vi "CSV_Setup_Data_Handler.vi"(0 "first iteration":bool, 1 "Timeout 1":bool, 7 "Sample Data":dbl[](array[numeric]), 9 "Sample Data 2":dbl[](array[numeric]), 11 "Data":T1={"Pinch-valve"="", "XLP 6000 Pump"="", "Camera1"="", "Camera2"="", "Img_Capt"=FALSE, "Actuator"=FALSE, "Pump"=FALSE, "Cam 1"=FALSE, "Cam 2"=FALSE, "Empty_Refill"=FALSE, "Crop"=FALSE, "Light intensity"=0, "Exposure Time"=0.0, "Sample Name"="", "Operator"="", "Calibration 1"=path "", "Calibration 2"=path "", "Framerate"=0, "Timeout Sample"=0, "Collection date"="", "Sample size threshold"=0, "Empty start"=0, "Command"="", "Station"="", "Species Name"="", "Other Notes"="", "Aperture"=enum."Item 0", "Image Process Queue Size"=0, "Image Save Queue Size"=0, "Overload threshold"=0, "Max Framerate"=0, "Rectangle 1"={"Left"=0, "Top"=0, "Right"=0, "Bottom"=0, "Rotation"=0.0}, "Rectangle 2"={"Left"=0, "Top"=100, "Right"=100, "Bottom"=0, "Rotation"=0.0}, "Detection Region %"=200.0, "Detect 1"=path "", "Detect 2"=path "", "Max large object threshold"=500, "Open(T)/Close(F)"=FALSE, "Img_Capt Begin"=FALSE, "Dispense Speed"=0, "Flush Size"=0, "Location"="", "Latitude"="", "Longitude"="", "Determiner"="", "Sex"="", "Camera1_Img"=refnum, "Camera2_Img"=refnum, "Img1_Orig_Disp"=refnum, "Img2_Orig_Disp"=refnum, "Img1_Orig_RGB"=refnum, "Img2_Orig_RGB"=refnum, "Blue_Plane_Extract"=refnum, "Subtracted_Plane"=refnum, "Img1_Binary"=refnum, "Img2_Binary"=refnum, "Crop_Mask"=refnum, "Img1_Save"=refnum, "Img2_Save"=refnum, "Img1_Cali_Full"=refnum, "Img2_Cali_Full"=refnum, "Img1_Cali_Detect"=refnum, "Img2_Cali_Detect"=refnum, "Cam 1 queue"=refnum, "Cam 2 queue"=refnum, "Cam 1 - save queue"=refnum, "Cam 2 - save queue"=refnum, "Overlay_Ring"=0, "SystemVersion"=0, "System Serial"="", "Legacy Cam Attributes"=FALSE, "Camera Orientation 1"="", "Camera Orientation 2"="", "Pixel to mm 1"=0.0, "Pixel to mm 2"=0.0, "CAM1 Model"=enum."a2A5328-15ucBAS", "CAM2 Model"=enum."a2A5328-15ucBAS", "Flush Insect"=FALSE, "Pump Size"=FALSE, "Barcode"="", "Phase3"=FALSE, "Mega F3"="", "Container nr."=0.0, "Flush Error"=TRUE, "Start System"=FALSE, "Size Interval"=0.0, "Mun. of containers"=0.0, "Sorting sys."=FALSE, "Initial size"=0.0} {"SystemVersion" items=["Standard", "XL"]; "Overlay_Ring" items=["Session Data", "Extended Setup", "Buffer", "Camera", "Dispenser", "Stats", "Connections"]; "Flush Size" min=1; "Dispense Speed" min=1; "Rectangle 2"."Rotation" format="%.2f"; "Rectangle 2"."Left" scale=0.0..1024.0; "Rectangle 2"."Right" scale=0.0..1024.0; "Rectangle 1"."Rotation" format="%.2f"; "Rectangle 1"."Left" scale=0.0..1024.0; "Rectangle 1"."Right" scale=0.0..1024.0; "Max Framerate" min=1; "Overload threshold" min=1; "Image Save Queue Size" min=1; "Image Process Queue Size" min=1; "Empty start" min=1; "Sample size threshold" min=1; "Framerate" min=1; "Light intensity" scale=0.0..100.0}, 12 "Timeout 2":bool) -> (4 "Sample Name":string, 6 "Ready file created":bool, 10 "Cam1_Stats":cluster{"Mean_Area":i32, "Img_Count":u32} caption="Camera 1", 14 "Container barcode":string, 15 "Cam2_Stats":cluster{"Mean_Area":i32, "Img_Count":u32} caption="Camera 2")   [LabVIEW 2024]
uses:
  controls/Data.ctl
  <vilib>/userDefined/High Color/IMAQdx.ctl
  <vilib>/vision/Image Controls.llb/IMAQ Image.ctl
panel:
  in  "Stop":bool
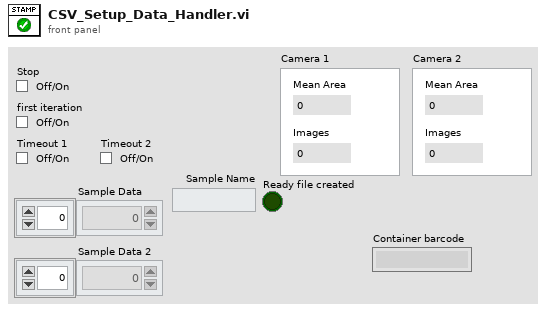
[diagram p1: front panel]
types:
  T1 = typedef "Data.ctl" = cluster{"Pinch-valve":refnum<visa-resource-name>, "XLP 6000 Pump":refnum<visa-resource-name>, "Camera1":T2, "Camera2":T2, "Img_Capt":bool, "Actuator":bool, "Pump":bool, "Cam 1":bool, "Cam 2":bool, "Empty_Refill":bool, "Crop":bool, "Light intensity":i32, "Exposure Time":dbl, "Sample Name":string, "Operator":string, "Calibration 1":path, "Calibration 2":path, "Framerate":i32, "Timeout Sample":i32, "Collection date":string, "Sample size threshold":i32, "Empty start":u32, "Command":string, "Station":string, "Species Name":string, "Other Notes":string, "Aperture":enum32{"Item 0", "Item 1", "Item 2", "Item 3"}, "Image Process Queue Size":i32, "Image Save Queue Size":i32, "Overload threshold":i32, "Max Framerate":i32, "Rectangle 1":T3, "Rectangle 2":T3, "Detection Region %":dbl, "Detect 1":path, "Detect 2":path, "Max large object threshold":i32, "Open(T)/Close(F)":bool, "Img_Capt Begin":bool, "Dispense Speed":i32, "Flush Size":i32, "Location":string, "Latitude":string, "Longitude":string, "Determiner":string, "Sex":string, "Camera1_Img":T4, "Camera2_Img":T4, "Img1_Orig_Disp":T4, "Img2_Orig_Disp":T4, "Img1_Orig_RGB":T4, "Img2_Orig_RGB":T4, "Blue_Plane_Extract":T4, "Subtracted_Plane":T4, "Img1_Binary":T4, "Img2_Binary":T4, "Crop_Mask":T4, "Img1_Save":T4, "Img2_Save":T4, "Img1_Cali_Full":T4, "Img2_Cali_Full":T4, "Img1_Cali_Detect":T4, "Img2_Cali_Detect":T4, "Cam 1 queue":refnum<queue>, "Cam 2 queue":refnum<queue>, "Cam 1 - save queue":refnum<queue>, "Cam 2 - save queue":refnum<queue>, "Overlay_Ring":u16, "SystemVersion":u16, "System Serial":string, "Legacy Cam Attributes":bool, "Camera Orientation 1":string, "Camera Orientation 2":string, "Pixel to mm 1":dbl, "Pixel to mm 2":dbl, "CAM1 Model":enum16{"a2A5328-15ucBAS", "acA1920-155uc"}, "CAM2 Model":enum16{"a2A5328-15ucBAS", "acA1920-155uc"}, "Flush Insect":bool, "Pump Size":bool, "Barcode":string, "Phase3":bool, "Mega F3":refnum<visa-resource-name>, "Container nr.":dbl, "Flush Error":bool, "Start System":bool, "Size Interval":dbl, "Mun. of containers":dbl, "Sorting sys.":bool, "Initial size":dbl}
  T2 = typedef "IMAQdx.ctl" = refnum<k21>
  T3 = typedef "IMAQ Rectangle" = cluster{"Left":i32, "Top":i32, "Right":i32, "Bottom":i32, "Rotation":dbl}
  T4 = typedef "IMAQ Image.ctl" = refnum<image>
  T5 = cluster{"MFD max":string, "MFD mean":string, "MFD std. dev.":string, "Perim. mean":string, "Perim. std. dev":string, "Area mean":string, "Area std. dev.":string, "Holes mean":string, "Holes std. dev.":string, "Area+Holes mean":string, "Area+Holes std. dev.":string}
  T6 = cluster{"MFD max":string, "MFD mean":string, "MFD std. dev.":string, "Perim. mean":string, "Perim. std. dev":string, "Area mean":string, "Area std. dev.":string, "Holes mean":string, "Holes std. dev.":string, "Area+Holes mean":string, "Area+Holes std. dev.":string, "Barcode":string}
  T7 = cluster{"MFD max":string, "MFD mean":string, "MFD std. dev.":string, "Perim. mean":string, "Perim. std. dev":string, "Area mean":string, "Area std. dev.":string, "Holes mean":string, "Holes std. dev.":string, "Area+Holes mean":string, "Area+Holes std. dev.":string, "Container barcode":string}
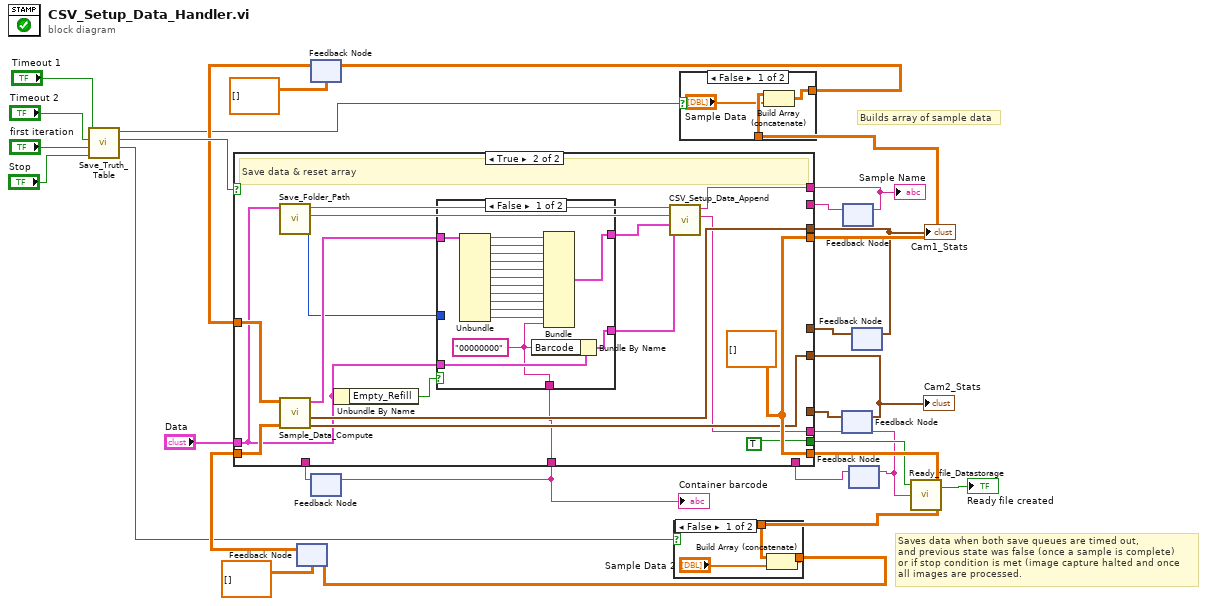
[diagram p0: block diagram]
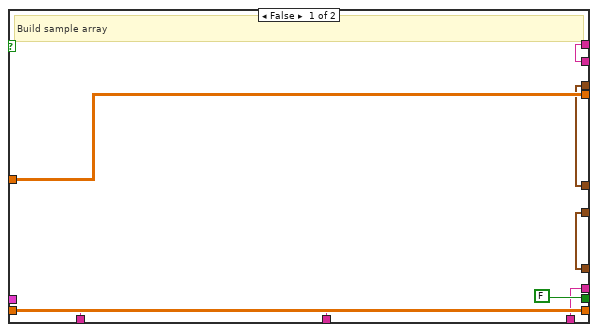
[diagram p4: hidden frame]
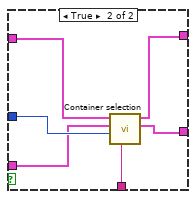
[diagram p5: hidden frame]
diagram:
  # "Builds array of sample data"
  # "Saves data when both save queues are timed out, \nand previous state was false (once a sample is complete)\nor if stop condition is met (image capture halted and once\nall images are processed."
  n1 = call "Save_Truth_Table.vi"("Stop"="Stop", "first iteration"="first iteration", "Timeout 2"="Timeout 2", "Timeout 1"="Timeout 1") -> ("Append Sample Data 2"=w18:bool, "Save_Data"=w21:bool, "Append Sample Data 1"=w19:bool)  [unwired: 5 in]
  n2 = feedback #1(dbl[][] []) -> (w24:dbl[][])
  n3 = feedback #2(dbl[][] []) -> (w20:dbl[][])
  n4 = feedback #3() -> (w1:string)  [unwired: 1 in]
  n5 = feedback #4() -> (w9:cluster{"Mean_Area":i32, "Img_Count":u32})  [unwired: 1 in]
  n6 = feedback #5() -> (w11:string)  [unwired: 1 in]
  n7 = feedback #6() -> (w4:string)  [unwired: 1 in]
  n8 = feedback #7() -> (w10:cluster{"Mean_Area":i32, "Img_Count":u32})  [unwired: 1 in]
  n9 = case shown="True" w21 {
    tunnel: "Data" -> [_ w39]
    tunnel: w24 -> [w36 w52]
    tunnel: [w36 w53] -> w22
    tunnel: w20 -> [w35 w51]
    tunnel: [w35 w53] -> w28
    tunnel: [w34 w48] -> w12
    tunnel: [w32 w47] -> w8
    tunnel: [w33 w46] -> w7
    tunnel: w11 -> [w34 _]
    tunnel: w10 -> [w33 _]
    tunnel: w9 -> [w32 _]
    tunnel: [FALSE TRUE] -> w6
    tunnel: [w30 w44] -> w5
    tunnel: w4 -> [w30 _]
    tunnel: [w29 w41] -> w2
    tunnel: w1 -> [w29 _]
    frame False {
      # "Build sample array"
    }
    frame True {
      w53 = dbl[][] []
      # "Save data & reset array"
      n10 = call "Save_Folder_Path.vi"("input cluster"=w39) -> ("Sample cnt."=w40:i32, "Subfolder Name"=w50:string, "Subfolder Path"=w49:string)  [unwired: 8 in]
      n11 = call "Sample_Data_Compute.vi"("Data Array 2"=w52, "Data Array 1"=w51) -> ("Cam2_Stats"=w47:cluster{"Mean_Area":i32, "Img_Count":u32}, "Cam1_Stats"=w46:cluster{"Mean_Area":i32, "Img_Count":u32}, "output cluster"=w42:T5)  [unwired: 6 in, 1 out]
      n12 = Unbundle By Name(w39) -> ("Empty_Refill"=w38:bool)
      n13 = case shown="False" w38 {
        tunnel: [w68 w75] -> w43
        tunnel: w42 -> [w67 w74]
        tunnel: [w54 w73] -> w37
        tunnel: [w55 w72] -> w41
        tunnel: w40 -> [_ w71]
        tunnel: w39 -> [w69 w70]
        frame False {
          w55 = "00000000" ("Barcode")
          n14 = Unbundle(w67) -> ("MFD max"=w66:string, "MFD mean"=w65:string, "MFD std. dev."=w64:string, "Perim. mean"=w63:string, "Perim. std. dev"=w62:string, "Area mean"=w61:string, "Area std. dev."=w60:string, "Holes mean"=w59:string, "Holes std. dev."=w58:string, "Area+Holes mean"=w57:string, "Area+Holes std. dev."=w56:string)
          n15 = Bundle By Name(cluster=w69, "Barcode"=w55) -> (w68:T1)
          n16 = Bundle("MFD max"=w66, "MFD mean"=w65, "MFD std. dev."=w64, "Perim. mean"=w63, "Perim. std. dev"=w62, "Area mean"=w61, "Area std. dev."=w60, "Holes mean"=w59, "Holes std. dev."=w58, "Area+Holes mean"=w57, "Area+Holes std. dev."=w56, "Barcode"=w55) -> (w54:T6)  [unwired: 1 in]
        }
        frame True {
          n17 = call "Container selection.vi"("Insect number"=w71, "Data"=w70, "Input cluster"=w74) -> ("Data Out"=w75:T1, "output cluster"=w73:T7, "Container barcode"=w72:string)  [unwired: 3 in, 3 out]
        }
      }
      n18 = call "CSV_Setup_Data_Append.vi"("input cluster"=w43, "Sample cluster"=w37, "Sample Name"=w50, "Image path"=w49) -> ("File Path"=w44:string, "Sample Name dup"=w48:string)  [unwired: 6 in]
    }
  }
  "Sample Name" <- w12
  "Cam1_Stats" <- w7
  "Cam2_Stats" <- w8
  "Container barcode" <- w2
  n19 = feedback-in #3(w2) -> ()
  n20 = case shown="False" w18 {
    tunnel: [w78 w79] -> w23
    tunnel: w22 -> [w77 w79]
    frame False {
      n21 = Build Array (concatenate)(w77, "Sample Data 2") -> (w78:dbl[][])
    }
    frame True {
    }
  }
  n22 = feedback-in #1(w23) -> ()
  n23 = case shown="False" w19 {
    tunnel: w28 -> [w82 w83]
    tunnel: [w81 w83] -> w25
    frame False {
      n24 = Build Array (concatenate)(w82, "Sample Data") -> (w81:dbl[][])
    }
    frame True {
    }
  }
  n25 = feedback-in #2(w25) -> ()
  n26 = feedback-in #4(w8) -> ()
  n27 = feedback-in #5(w12) -> ()
  n28 = feedback-in #6(w5) -> ()
  n29 = feedback-in #7(w7) -> ()
  n30 = call "Ready_file_Datastorage.vi"("File Path"=w5, "File save"=w6) -> ("Ready file created"=→"Ready file created":bool)  [unwired: 2 in]
